vi "Handle Events.vi"(8 "error in (no error)":errorcluster, 11 "MenuButton Event Handler in":refnum<class "MenuButton Event Handler.lvclass">) -> ()   [LabVIEW 2017, in "MenuButtons.lvlib" / "MenuButton Event Handler.lvclass"]
uses:
  MenuButton Event Handler.lvclass
  MenuButton Event Handler.lvclass/MenuButton Event Handler.ctl
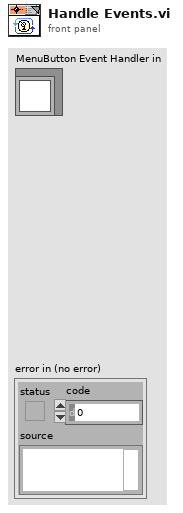
[diagram p1: front panel]
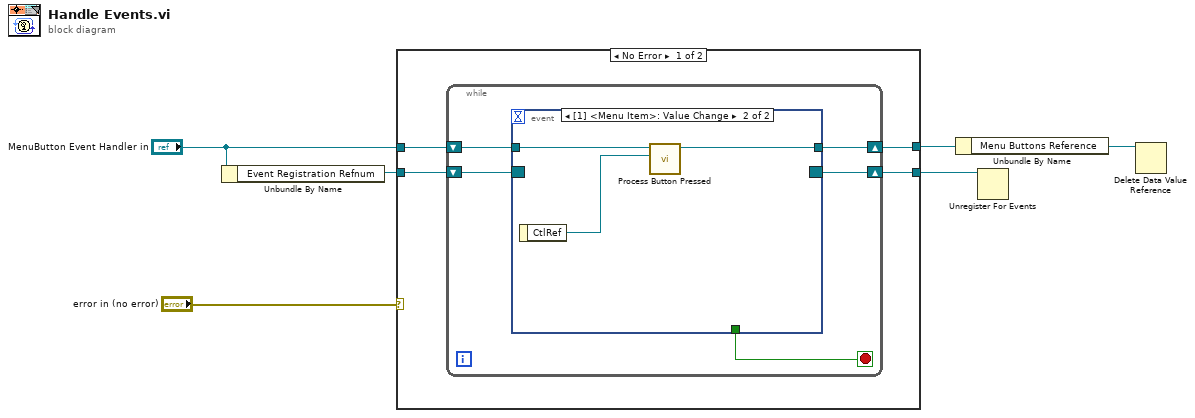
[diagram p0: block diagram]
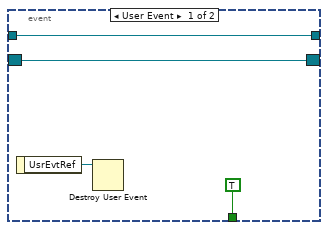
[diagram p2: hidden frame]
diagram:
  n1 = Unbundle By Name("MenuButton Event Handler in") -> ("Event Registration Refnum"=w4:refnum<event-registration>)
  n2 = case shown="No Error" "error in (no error)" {
    tunnel: "MenuButton Event Handler in" -> [w10 w23]
    tunnel: w4 -> [w9 w24]
    tunnel: [w8 w24] -> w3
    tunnel: [w7 w23] -> w2
    frame No Error {
      n3 = while {
        shift-right: [w13] -> w7
        shift-left: w10 -> [w14]
        shift-right: [w12] -> w8
        shift-left: w9 -> [w15]
        stop <- w11 stop-if-true
        n4 = event shown="[1] <Menu Item>: Value Change" {
          selector: w15 -> [w16 _]
          dyn-events: [w16 _] -> w12
          timeout: _ -> [_ _]
          tunnel: w14 -> [w17 w22]
          tunnel: [w17 w21] -> w13
          tunnel: [TRUE _] -> w11
          event User Event {
            n5 = event-data() -> ("UsrEvtRef"=w18:refnum<user-event>)  [unwired: 1 in]
            n6 = Destroy User Event(user event=w18) -> ()  [unwired: 1 in, 1 out]
          }
          event Value Change {
            n7 = event-data() -> ("CtlRef"=w20:refnum<vi>)  [unwired: 1 in]
            n8 = call "Process Button Pressed.vi"("Menu Reference"=w20, "MenuButton Event Handler in"=w22) -> ("MenuButton Event Handler out"=w21:refnum<class "MenuButton Event Handler.lvclass">)  [unwired: 8 in, 1 out]
          }
        }
      }
    }
    frame Error {
    }
  }
  n9 = Unbundle By Name(w2) -> ("Menu Buttons Reference"=w1:refnum<data-value>)
  n10 = Unregister For Events(event registration refnum=w3) -> ()  [unwired: 1 in, 1 out]
  n11 = Delete Data Value Reference(data value reference=w1) -> ()  [unwired: 1 in, 2 out]
